vi "Connect (PuTTY).vi"(6 "timeout (ms)":i32=30000, 8 "error in":errorcluster, 10 "user@host":string, 11 "client":refnum<class "PuTTY Client.lvclass">) -> (0 "error out":errorcluster, 3 "session":refnum<class "Session.lvclass">)   [LabVIEW 2020, in "NI_SFTP.lvlib"]
doc: "Connects to an SFTP server using the Plink executable typically installed with the PuTTY client."
uses:
  <vilib>/net/SFTP/NI_SFTP.lvlib
  <vilib>/net/SFTP/Session/Session.lvclass
  <vilib>/net/SSH/Client/PuTTY/PuTTY Client.lvclass
  e:/builds/penguin/labview/branches/2020/dev/dist/vi.lib/net/SSH/Client/Generic/Generic Client.lvclass
  <vilib>/net/SFTP/Session/Session.lvclass/Session.ctl
  <vilib>/net/SFTP/Session/Write SSH Client.vi
  <vilib>/net/SFTP/Session/Write user_host.vi
  <vilib>/Utility/Deadline/NI_Deadline.lvlib
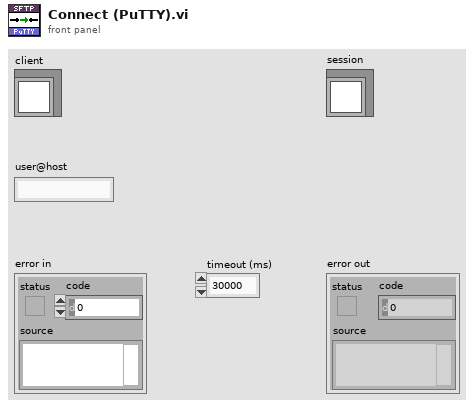
[diagram p1: front panel]
types:
  T1 = typedef "NI_Deadline.lvlib/Deadline.ctl" = cluster{"mode":T2, "deadline (ms)":u32}
  T2 = typedef "NI_Deadline.lvlib/Mode.ctl" = enum16{"Relative", "Use deadline", "Wait forever", "Nonblocking", "N/A"}
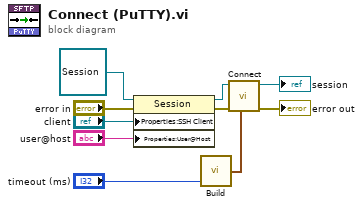
[diagram p0: block diagram]
diagram:
  n1 = property class="Session"(reference=refnum<class "Session.lvclass"> refnum ("Session in"), error in="error in", "Properties:SSH Client"="client", "Properties:User@Host"="user@host") -> (reference out=w9:refnum<class "Session.lvclass">, error out=w7:errorcluster)
  n2 = call <vilib>:"Build.vi"("timeout (ms)"="timeout (ms)") -> ("Deadline out"=w8:T1)  [unwired: 2 in]
  n3 = call-dynamic "Connect.vi"("deadline"=w8, "error in"=w7, "session in"=w9) -> ("error out"=→"error out":errorcluster, "session out"=→"session":refnum<class "Session.lvclass">)  [unwired: 7 in]
